vi "Open EXE.vi"(0 "command line":string) -> ()   [LabVIEW 2015]
panel:
  in  "wait until completion?":bool
  in  "Path":path
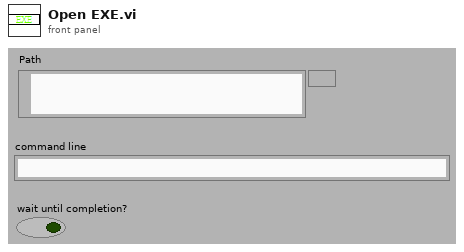
[diagram p1: front panel]
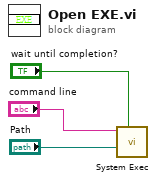
[diagram p0: block diagram]
diagram:
  n1 = call <vilib>:"System Exec.vi"("wait until completion? (T)"="wait until completion?", "working directory"="Path", "command line"="command line") -> ()  [unwired: 5 in, 4 out]
